vi "UTILITY Get Last Dataset.vi"(11 "Full Dataset":string[][](array[string])) -> (3 "Last Recorded Dataset":string[][](array[string]))   [LabVIEW 2020]
panel:
  out "Header":string[](array[string])
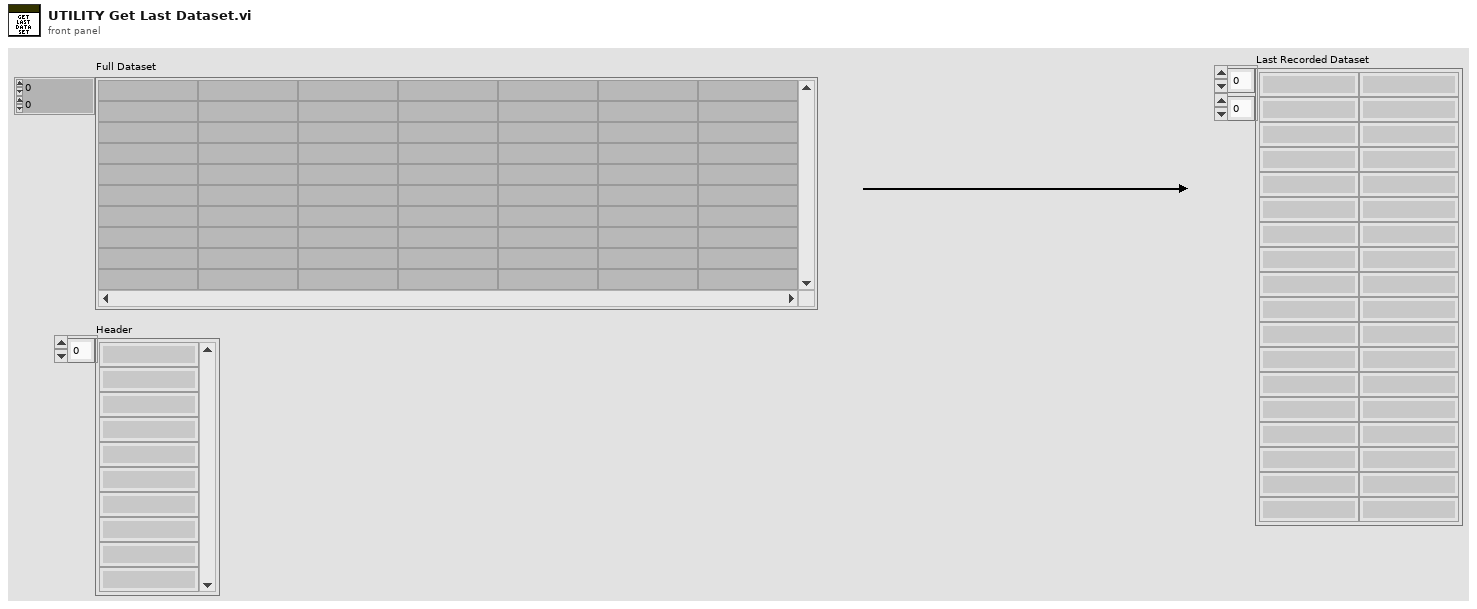
[diagram p1: front panel]
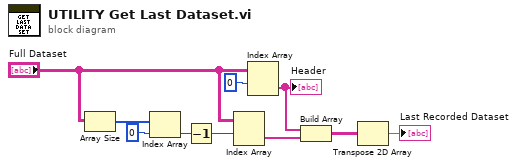
[diagram p0: block diagram]
diagram:
  n1 = Array Size(array="Full Dataset") -> (size(s)=w10:i32[])
  n2 = Index Array(array=w10, index=0) -> (element=w8:i32)
  n3 = Decrement(x=w8) -> (x-1=w7:i32)
  n4 = Index Array(array="Full Dataset", index (row)=w7) -> (element=w6:string[])  [unwired: 1 in]
  n5 = Index Array(array="Full Dataset", index (row)=0 ("disabled index (col)")) -> (element=w1:string[])  [unwired: 1 in]
  "Header" <- w1
  n6 = Build Array(w1, w6) -> (w5:string[][])
  n7 = Transpose 2D Array(2D array=w5) -> (transposed array=→"Last Recorded Dataset":string[][])
